vi "Pixel_integrator.vi"(8 "Pixels to integrate":i32, 9 "Data in":dbl[](array[numeric])) -> (2 "Leftover data out":dbl[](array[numeric]), 3 "Data out":dbl[](array[numeric]))   [LabVIEW 2010]
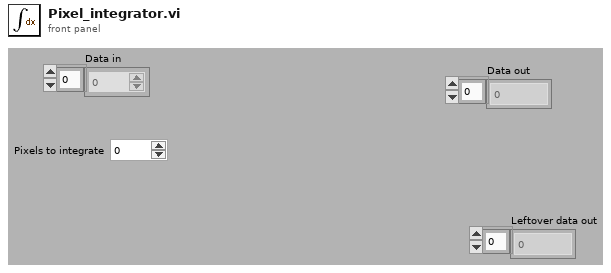
[diagram p1: front panel]
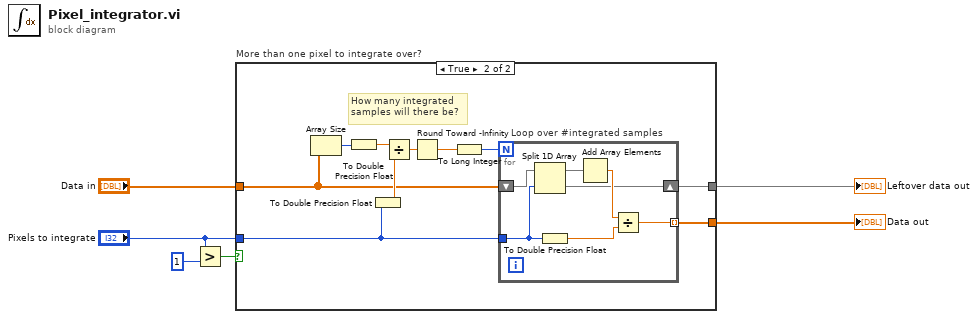
[diagram p0: block diagram]
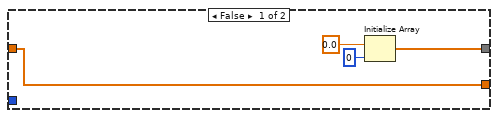
[diagram p2: hidden frame]
diagram:
  n1 = Greater?(x="Pixels to integrate", y=1) -> (0:w1:bool)
  n2 = case "More than one pixel to integrate over?" shown="True" w1 {
    tunnel: [w8 w12] -> w4
    tunnel: "Data in" -> [w7 w13]
    tunnel: "Pixels to integrate" -> [_ w15]
    tunnel: [w7 w11] -> w3
    frame False {
      n3 = Initialize Array(0.0 ("element"), 0 ("dimension size")) -> (w8:dbl[])
    }
    frame True {
      # "How many integrated\nsamples will there be?"
      n4 = Array Size(array=w13) -> (size(s)=w16:i32)
      n5 = To Double Precision Float(number=w16) -> (double precision float=w19:dbl)
      n6 = To Double Precision Float(number=w15) -> (double precision float=w14:dbl)
      n7 = Divide(x=w19, y=w14) -> (x/y=w20:dbl)
      n8 = Round Toward -Infinity(1:w20) -> (0:w18:dbl)
      n9 = To Long Integer(number=w18) -> (32bit integer=w17:i32)
      n10 = for "Loop over #integrated samples" {
        N: w17 -> [_]
        tunnel: w15 -> [w23]
        shift-right: [w21] -> w12
        shift-left: w13 -> [w24]
        tunnel: [w25] -> w11 mode=indexing
        n11 = Split 1D Array(array=w24, index=w23) -> (first subarray=w22:dbl[], second subarray=w21:dbl[])
        n12 = To Double Precision Float(number=w23) -> (double precision float=w26:dbl)
        n13 = Add Array Elements(numeric array=w22) -> (sum=w27:dbl)
        n14 = Divide(x=w27, y=w26) -> (x/y=w25:dbl)
      }
    }
  }
  "Data out" <- w3
  "Leftover data out" <- w4
